vi "Read Icon.vi"(8 "error in (no error)":errorcluster, 11 "TTLDevice in":refnum<class "TTLControlledDevice.lvclass">) -> (0 "error out":errorcluster, 2 "Icon":picture, 3 "TTLDevice out":refnum<class "TTLControlledDevice.lvclass">)   [LabVIEW 2015, in "TTLControlledDevice.lvclass"]
uses:
  TTLControlledDevice.lvclass
panel:
  out "Water":picture
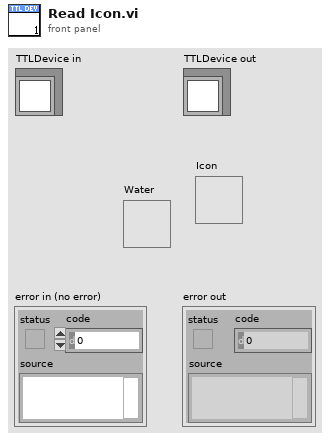
[diagram p1: front panel]
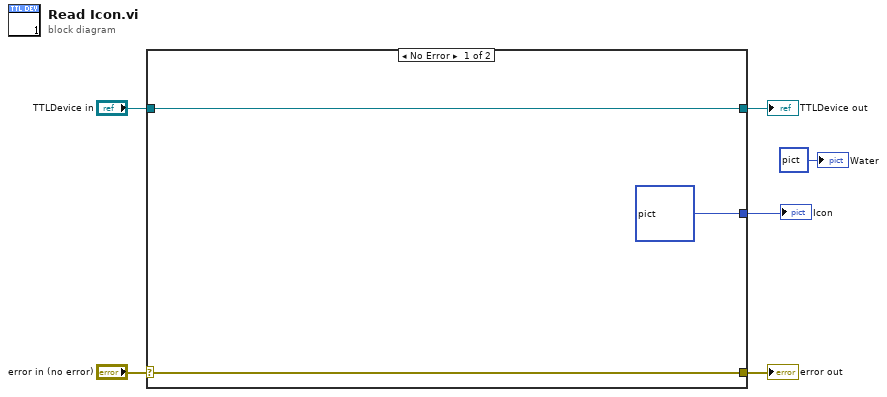
[diagram p0: block diagram]
diagram:
  n1 = case shown="No Error" "error in (no error)" {
    selector: "error in (no error)" -> [w8 w11]
    tunnel: [w8 w11] -> w5
    tunnel: [w9 w10] -> w3
    tunnel: "TTLDevice in" -> [w9 w10]
    tunnel: [picture bytes[7230] ("Icon") _] -> w1
    frame No Error {
    }
    frame Error {
    }
  }
  "error out" <- w5
  "TTLDevice out" <- w3
  "Icon" <- w1
  "Water" <- picture bytes[7230] ("Water")
